vi "update Status String.vi"(8 "error in (no error)":errorcluster, 10 "Data to Append":string, 11 "Import Export SQL in":refnum<class "Import Export SQL.lvclass">) -> (0 "error out":errorcluster, 3 "Import Export SQL out":refnum<class "Import Export SQL.lvclass">)   [LabVIEW 2023, in "Data Analysis.lvlib" / "Import Export SQL.lvlib" / "Import Export SQL.lvclass"]
uses:
  Import Export SQL.lvclass
  Import Export SQL.lvclass/Import Export SQL.ctl
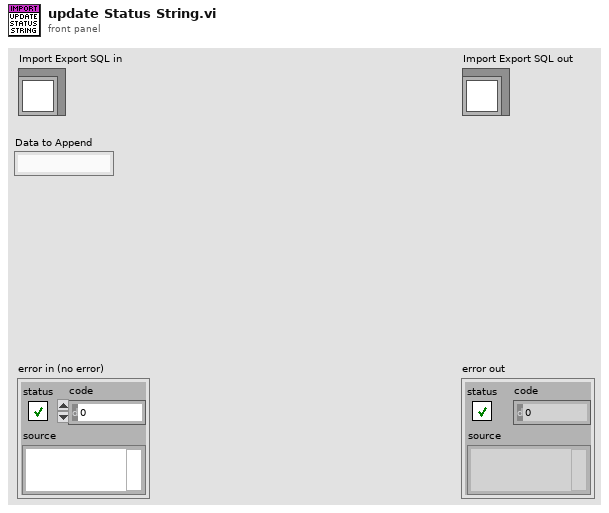
[diagram p1: front panel]
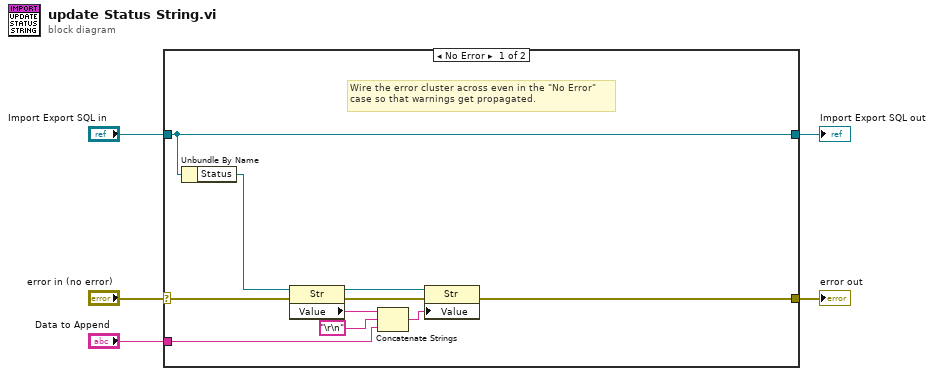
[diagram p0: block diagram]
diagram:
  n1 = case shown="No Error" "error in (no error)" {
    selector: "error in (no error)" -> [w14 w17]
    tunnel: [w6 w17] -> w4
    tunnel: [w15 w16] -> w2
    tunnel: "Import Export SQL in" -> [w15 w16]
    tunnel: "Data to Append" -> [w8 _]
    frame No Error {
      # "Wire the error cluster across even in the \"No Error\"\ncase so that warnings get propagated."
      n2 = Unbundle By Name(w15) -> ("Status"=w13:refnum<vi>)
      n3 = property class="Str"(reference=w13, error in=w14) -> (reference out=w12:refnum<vi>, error out=w11:errorcluster, "Value"=w10:string)
      n4 = Concatenate Strings(w10, "\r\n", w8) -> (w7:string)
      n5 = property class="Str"(reference=w12, error in=w11, "Value"=w7) -> (error out=w6:errorcluster)  [unwired: 1 out]
    }
    frame Error {
    }
  }
  "error out" <- w4
  "Import Export SQL out" <- w2
